vi "AI.vi"(2 "input array":u32[](array[numeric])) -> (0 "output array":u32[][](array[numeric]))   [LabVIEW 2020]
panel:
  out "return_snake":i32[](array[numeric])
  out "snake":u32[](array[numeric])
  out "food":i32
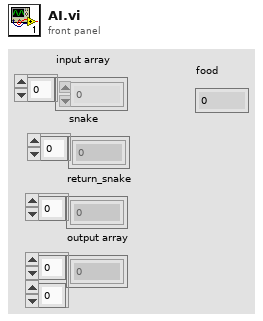
[diagram p1: front panel]
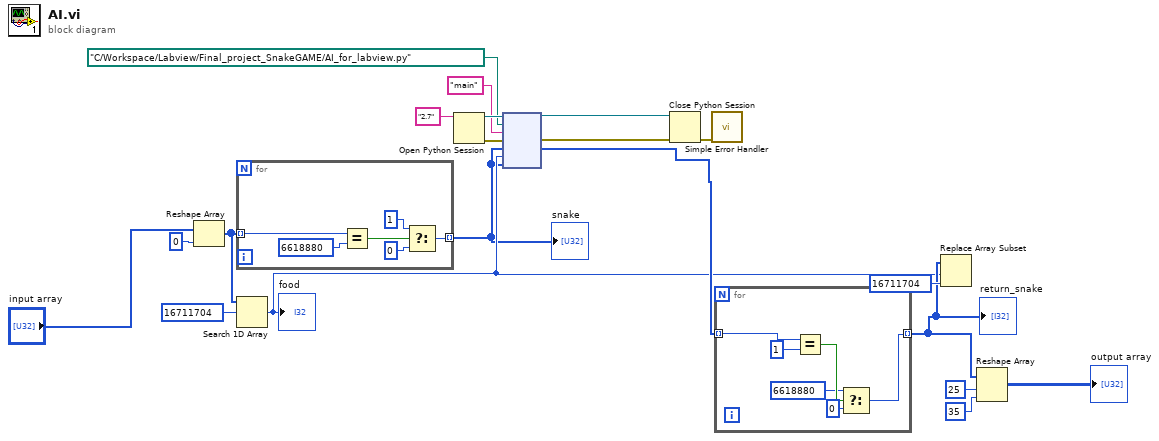
[diagram p0: block diagram]
diagram:
  n1 = Reshape Array("input array", 0 ("dimension size")) -> (w18:u32[])
  n2 = for {
    tunnel: w18 -> [w26] mode=indexing
    tunnel: [w21] -> w1 mode=indexing
    n3 = Equal?(x=w26, y=u32 6618880) -> (x = y?=w24:bool)
    n4 = Select(t=1, s=w24, f=0) -> (s? t:f=w21:i32)
  }
  "snake" <- w1
  n5 = Search 1D Array(1D array=w18, element=u32 16711704) -> (index of element=w2:i32)  [unwired: 1 in]
  "food" <- w2
  n6 = Open Python Session(python version="2.7" ("Python version")) -> (session out=w16:refnum<k35>, error out=w13:errorcluster)  [unwired: 2 in]
  n7 = node(w16, path "C:/Workspace/Labview/Final_project_SnakeGAME/AI_for_labview.py" ("module path"), "main" ("function name"), w13, w1, w2, w1) -> (w12:refnum<k35>, w11:errorcluster, w3:i32[])  [unwired: 2 in, 2 out]
  n8 = Close Python Session(session in=w12, error in=w11) -> (11:w10:errorcluster)
  n9 = call <vilib>:"Simple Error Handler.vi"("error in (no error)"=w10) -> ()  [unwired: 4 in, 5 out]
  n10 = for {
    tunnel: [w27] -> w8 mode=indexing
    tunnel: w3 -> [w32] mode=indexing
    n11 = Equal?(x=w32, y=1) -> (x = y?=w30:bool)
    n12 = Select(t=u32 6618880, s=w30, f=u32 0) -> (s? t:f=w27:u32)
  }
  "return_snake" <- w8
  n13 = Replace Array Subset(array=w8, new element=u32 16711704 ("new element/subarray"), index=w2) -> ()  [unwired: 1 out]
  n14 = Reshape Array(w8, 25 ("dimension size"), 35 ("dimension size")) -> (→"output array":u32[][])
